vi "Detener_Eje.vi"() -> ()   [LabVIEW 2017]
uses:
  <vilib>/Platform/TimedLoop/XDataNode/timing_clust.ctl
  <vilib>/Platform/TimedLoop/XDataNode/nitl_modes.ctl
  <vilib>/Platform/TimedLoop/XDataNode/wakeup.ctl
  <vilib>/Motion/Express/_s/nimc.fb.stopMove.stop.axis.modeDecelerate.vi
  <vilib>/Motion/Express/_s/nimc.fb.stopMove.stop.axis.modeImmediate.vi
  <vilib>/Motion/Express/_s/nimc.fb.stopMove.stop.axis.modeDeactivate.vi
  <vilib>/platform/TimedLoop/XDataNode/XDataNode.xnode
  <vilib>/Motion/BlockNode/FB.NIMotion.xnode
  <vilib>/Platform/TimedLoop/XDataNode/XDNodeRunTimeDep.lvlib
panel:
  in  "Opciones":T1(ring)
  out "done":bool
  in  "execute":bool
  in  "resource":refnum<k21>
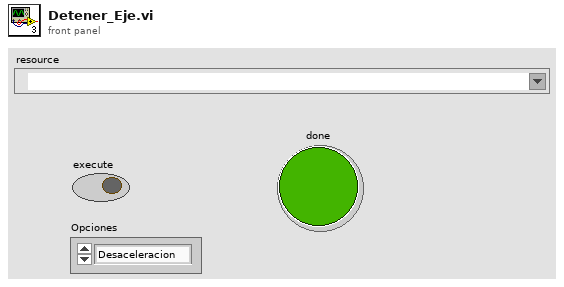
[diagram p1: front panel]
types:
  T1 = enum16{"Desaceleracion", "Inmediata", "Deshabilitar"}
  T2 = typedef "XDNodeRunTimeDep.lvlib/timing_clust.ctl" = cluster{"Expected End [f-1]":u64, "Actual End [f-1]":u64, "Finished Late? [f-1]":bool, "Expected End [i-1]":u64, "Actual End [i-1]":u64, "Finished Late? [i-1]":bool, "Expected Start [i]":u64, "Actual Start [i]":u64, "Expected Start [f]":u64, "Actual Start [f]":u64, "Source Name":string, "Structure Name":string, "Period":i64, "Deadline":i64, "Offset":i64, "Start":i64, "Priority":i32, "Timeout":i32, "Mode":T3, "Wakeup Reason":T4, "Error":errorcluster, "Source Type":string, "Secondary Source Type":string, "Global End Time":u64, "Global Start Time":u64, "Frame Duration":u64, "Iteration Duration":u64, "Assigned CPU":i32, "I/O Scan Engine Mode":u32}
  T3 = typedef "XDNodeRunTimeDep.lvlib/nitl_modes.ctl" = enum32{"No Change", "Process missed periods, maintain original phase", "Discard missed periods, maintain original phase", "Process missed periods, ignore original phase", "Discard missed periods, ignore original phase"}
  T4 = typedef "XDNodeRunTimeDep.lvlib/wakeup.ctl" = enum32{"Normal", "Aborted", "Asynchronous wakeup", "Timing source error", "Timed loop error", "Timeout"}
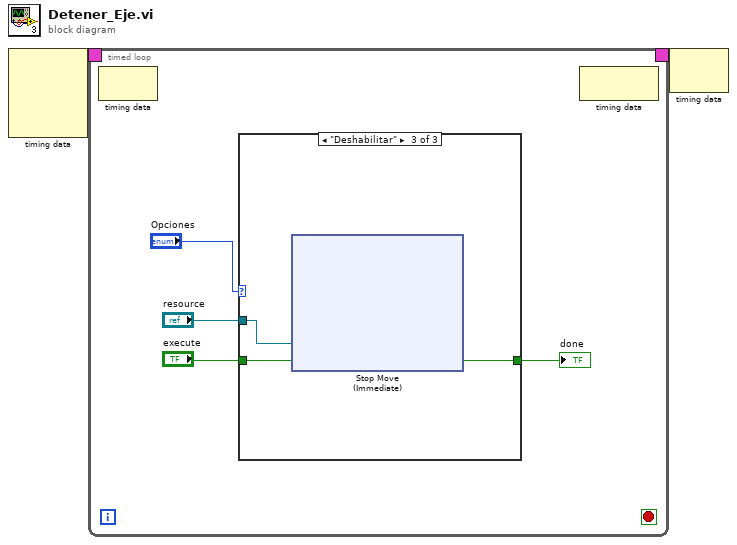
[diagram p0: block diagram]
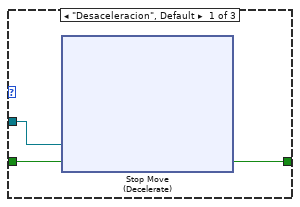
[diagram p2: hidden frame]
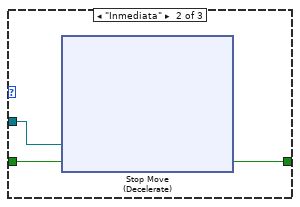
[diagram p3: hidden frame]
diagram:
  n1 = node-c288() -> (w2:T2)  [unwired: 4 in]
  n2 = timed-loop {
    timing: w2 -> [_]
    timing-out: [_] -> w1
    stop <- _ stop-if-true
    n3 = node-c288() -> ()  [unwired: 1 in, 1 out]
    n4 = case shown="\"Deshabilitar\"" "Opciones" {
      tunnel: "resource" -> [w9 w22 w35]
      tunnel: "execute" -> [w8 w21 w34]
      tunnel: [w7 w20 w33] -> w3
      frame "Desaceleracion", Default {
        n5 = xnode "Stop Move\n(Decelerate)"("resource"=w9, "execute"=w8) -> ("done"=w7:bool)  [unwired: 1 in, 2 out]
      }
      frame "Inmediata" {
        n6 = xnode "Stop Move\n(Decelerate)"("resource"=w22, "execute"=w21) -> ("done"=w20:bool)  [unwired: 1 in, 2 out]
      }
      frame "Deshabilitar" {
        n7 = xnode "Stop Move\n(Immediate)"("resource"=w35, "execute"=w34) -> ("done"=w33:bool)  [unwired: 1 in, 2 out]
      }
    }
    "done" <- w3
    n8 = node-c288() -> ()  [unwired: 1 in, 1 out]
  }
  n9 = node-c288(w1) -> ()  [unwired: 1 out]
